vi "Lockin to DAQ SMO config.vi"(8 "error in (no error)":errorcluster, 9 "SamplingInfo":cluster{"Fs":dbl, "#S":i32}={"Fs"=1000.0, "#S"=1000}, 10 "AO Configuration":T7, 11 "AI Configuration":T10) -> (0 "error out":errorcluster, 2 "DAQ_Manager.setDAQConfig":T1 {"DAQmx.AI.config"."input terminal configuration" items=["default"=-1, "RSE"=10083, "NRSE"=10078, "Differential"=10106, "Pseudodifferential"=12529]; "DAQmx.AI.config"."AI.Coupling" items=["AC"=10045, "DC"=10050, "GND"=10066]; "DAQmx.AO.config"."output terminal configuration" items=["Default"=-1, "RSE"=10083, "Differential"=10106, "Pseudodifferential"=12529]})   [LabVIEW 2019]
uses:
  SMOs/DAQmx.AI/Typedefs/AI.Terminal-enum.ctl
  SMOs/DAQmx.AO/Typedefs/AO.Terminal-enum.ctl
  SMOs/DAQmx.AI/Typedefs/AI.Coupling-enum.ctl
  SMOs/DAQmx.AO/Typedefs/DAQmx.AO_Config.ctl
  SMOs/DAQmx.AI/Typedefs/DAQmx.AI_Config.ctl
  SMOs/DAQ_Manager/Typedefs/PrivateEvents--DAQ_Manager.setDAQConfig.ctl
  Typedefs/446xAO-enum.ctl
  Typedefs/AO.config-cluster.ctl
  Typedefs/AO.config-array.ctl
  Typedefs/AI.coupling-enum.ctl
  Typedefs/446xAI-enum.ctl
  Typedefs/AI.config-cluster.ctl
  Typedefs/AI.config-array.ctl
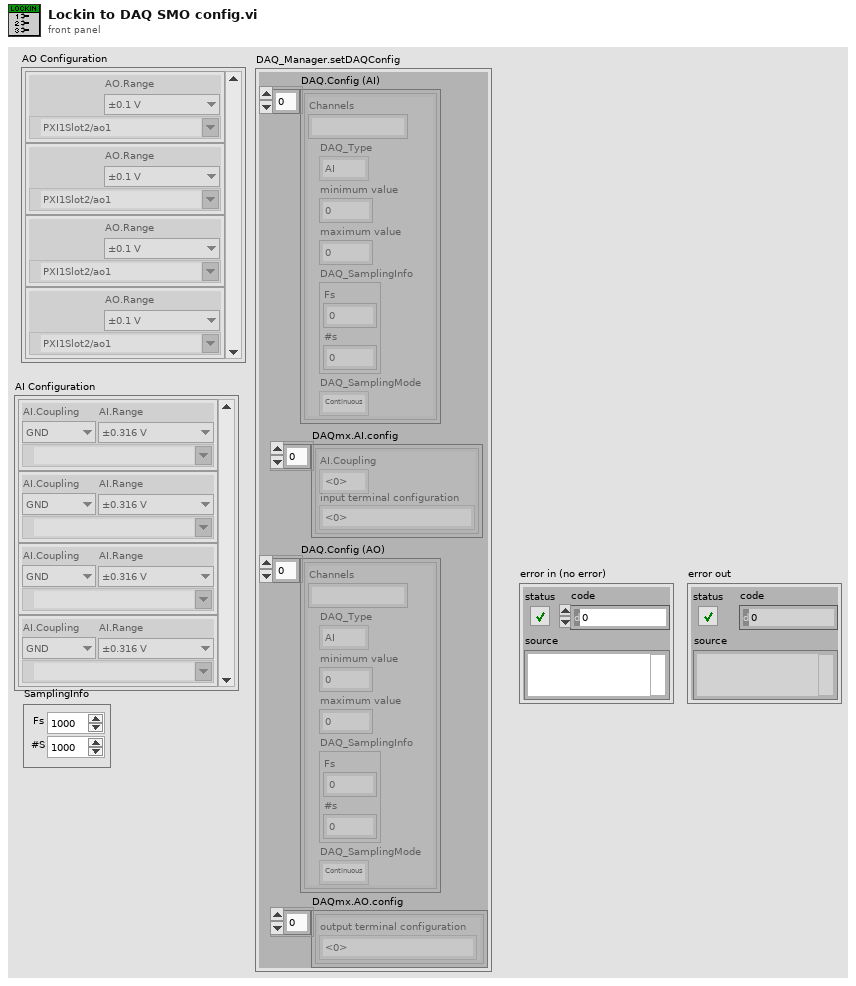
[diagram p1: front panel]
types:
  T1 = typedef "DAQ_Manager.lvclass/PrivateEvents--DAQ_Manager.setDAQConfig.ctl" = cluster{"DAQ.Config (AI)":cluster{"Channels":string, "DAQ_Type":enum16{"AI", "AO"}, "minimum value":dbl, "maximum value":dbl, "DAQ_SamplingInfo":cluster{"Fs":dbl, "#s":i32}, "DAQ_SamplingMode":enum16{"Continuous", "Finite"}}[], "DAQmx.AI.config":T2[], "DAQ.Config (AO)":cluster{"Channels":string, "DAQ_Type":enum16{"AI", "AO"}, "minimum value":dbl, "maximum value":dbl, "DAQ_SamplingInfo":cluster{"Fs":dbl, "#s":i32}, "DAQ_SamplingMode":enum16{"Continuous", "Finite"}}[], "DAQmx.AO.config":T5[]}
  T2 = typedef "DAQmx.AI.lvclass/DAQmx.AI_Config.ctl" = cluster{"AI.Coupling":T3, "input terminal configuration ":T4}
  T3 = typedef "DAQmx.AI.lvclass/AI.Coupling-enum.ctl" = i32
  T4 = typedef "DAQmx.AI.lvclass/AI.Terminal-enum.ctl" = i32
  T5 = typedef "DAQmx.AO.lvclass/DAQmx.AO_Config.ctl" = cluster{"output terminal configuration":T6}
  T6 = typedef "DAQmx.AO.lvclass/AO.Terminal-enum.ctl" = i32
  T7 = typedef "AO.config-array.ctl" = T8[]
  T8 = typedef "AO.config-cluster.ctl" = cluster{"AO.Range":T9, "AO.channels":tag}
  T9 = typedef "446xAO-enum.ctl" = enum16{"±0.1 V", "±1.0 V", "±10.0 V"}
  T10 = typedef "AI.config-array.ctl" = T11[]
  T11 = typedef "AI.config-cluster.ctl" = cluster{"AI.Coupling":T12, "AI.channels":tag, "AI.Range":T13}
  T12 = typedef "AI.coupling-enum.ctl" = enum16{"AC", "DC", "GND"}
  T13 = typedef "446xAI-enum.ctl" = enum16{"±0.316 V", "±1.00 V", "±3.16 V", "±10.0 V", "±31.6 V", "±42.4 V"}
  T14 = cluster{"Channels":string, "DAQ_Type":enum16{"AI", "AO"}, "minimum value":dbl, "maximum value":dbl, "DAQ_SamplingInfo":cluster{"Fs":dbl, "#s":i32}, "DAQ_SamplingMode":enum16{"Continuous", "Finite"}}[]
  T15 = cluster{"Channels":string, "DAQ_Type":enum16{"AI", "AO"}, "minimum value":dbl, "maximum value":dbl, "DAQ_SamplingInfo":cluster{"Fs":dbl, "#s":i32}, "DAQ_SamplingMode":enum16{"Continuous", "Finite"}}
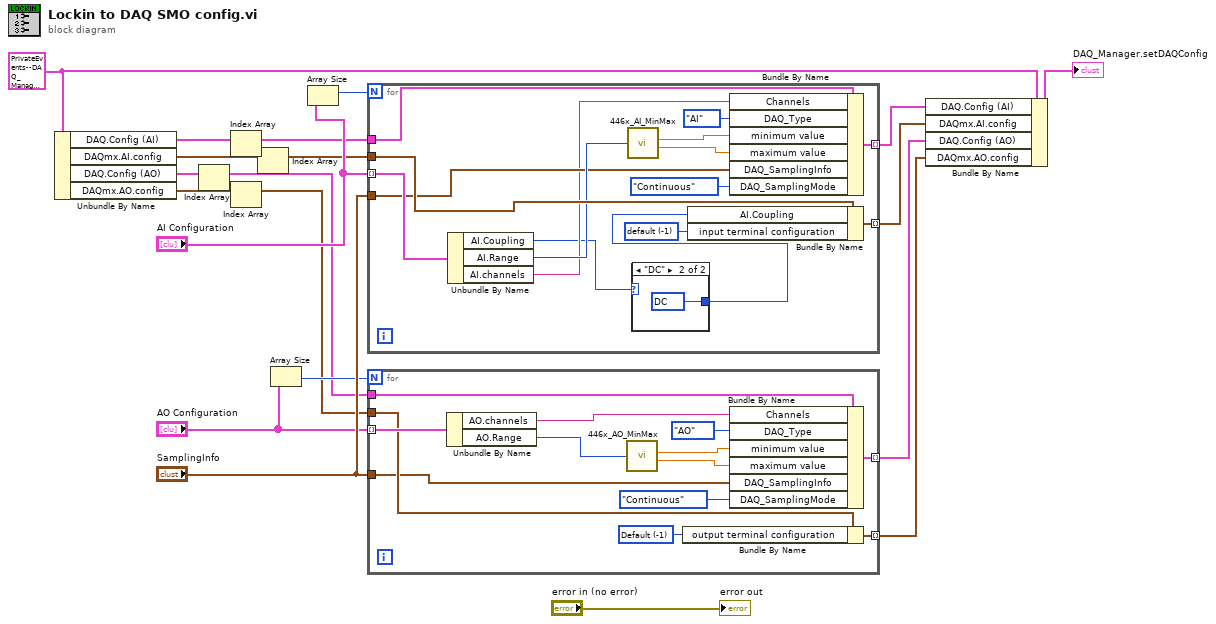
[diagram p0: block diagram]
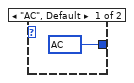
[diagram p2: hidden frame]
diagram:
  w2 = T1 {"DAQ.Config (AI)"=[{"Channels"="", "DAQ_Type"=enum."AI", "minimum value"=0.0, "maximum value"=0.0, "DAQ_SamplingInfo"={"Fs"=0.0, "#s"=0}, "DAQ_SamplingMode"=enum."Continuous"}], "DAQmx.AI.config"=[{"AI.Coupling"=10045, "input terminal configuration "=-1}], "DAQ.Config (AO)"=[{"Channels"="", "DAQ_Type"=enum."AI", "minimum value"=0.0, "maximum value"=0.0, "DAQ_SamplingInfo"={"Fs"=0.0, "#s"=0}, "DAQ_SamplingMode"=enum."Continuous"}], "DAQmx.AO.config"=[{"output terminal configuration"=-1}]} ("DAQ_Manager.setDAQConfig")
  n1 = Unbundle By Name(w2) -> ("DAQ.Config (AI)"=w17:T14, "DAQmx.AI.config"=w18:T2[], "DAQ.Config (AO)"=w19:T14, "DAQmx.AO.config"=w20:T5[])
  n2 = Index Array(array=w19) -> (element=w3:T15)  [unwired: 1 in]
  n3 = Index Array(array=w17) -> (element=w6:T15)  [unwired: 1 in]
  n4 = Index Array(array=w20) -> (element=w4:T5)  [unwired: 1 in]
  n5 = Index Array(array=w18) -> (element=w5:T2)  [unwired: 1 in]
  n6 = Array Size(array="AO Configuration") -> (size(s)=w9:i32)
  n7 = Array Size(array="AI Configuration") -> (size(s)=w7:i32)
  n8 = for {
    N: w7 -> [_]
    tunnel: w6 -> [w34]
    tunnel: w5 -> [w33]
    tunnel: "AI Configuration" -> [w35] mode=indexing
    tunnel: "SamplingInfo" -> [w28]
    tunnel: [w24] -> w14 mode=indexing
    tunnel: [w23] -> w13 mode=indexing
    w30 = T4 -1 items=["default"=-1, "RSE"=10083, "NRSE"=10078, "Differential"=10106, "Pseudodifferential"=12529] ("input terminal configuration")
    n9 = Unbundle By Name(w35) -> ("AI.Coupling"=w22:T12, "AI.Range"=w31:T13, "AI.channels"=w26:tag)
    n10 = call "446x_AI_MinMax.vi"("446x AI"=w31) -> ("AI.Min"=w32:dbl, "AI.Max"=w25:dbl)  [unwired: 6 in]
    n11 = case shown="\"DC\"" w22 {
      tunnel: [w36 w37] -> w21
      frame "AC", Default {
        w36 = T3 10045 items=["AC"=10045, "DC"=10050, "GND"=10066] ("AI.Coupling")
      }
      frame "DC" {
        w37 = T3 10050 items=["AC"=10045, "DC"=10050, "GND"=10066] ("AI.Coupling")
      }
    }
    n12 = Bundle By Name(cluster=w33, "AI.Coupling"=w21, "input terminal configuration"=w30) -> (w23:T2)
    n13 = Bundle By Name(cluster=w34, "Channels"=w26, "DAQ_Type"=enum16{"AI", "AO"}."AI", "minimum value"=w32, "maximum value"=w25, "DAQ_SamplingInfo"=w28, "DAQ_SamplingMode"=enum16{"Continuous", "Finite"}."Continuous") -> (w24:T15)
  }
  n14 = for {
    N: w9 -> [_]
    tunnel: w3 -> [w49]
    tunnel: w4 -> [w48]
    tunnel: "AO Configuration" -> [w50] mode=indexing
    tunnel: "SamplingInfo" -> [w45]
    tunnel: [w40] -> w12 mode=indexing
    tunnel: [w39] -> w11 mode=indexing
    w47 = T6 -1 items=["Default"=-1, "RSE"=10083, "Differential"=10106, "Pseudodifferential"=12529] ("output terminal configuration")
    n15 = Unbundle By Name(w50) -> ("AO.channels"=w41:tag, "AO.Range"=w38:T9)
    n16 = call "446x_AO_MinMax.vi"("AO.Range"=w38) -> ("AO.min"=w43:dbl, "AO.max"=w42:dbl)  [unwired: 6 in]
    n17 = Bundle By Name(cluster=w48, "output terminal configuration"=w47) -> (w39:T5)
    n18 = Bundle By Name(cluster=w49, "Channels"=w41, "DAQ_Type"=enum16{"AI", "AO"}."AO", "minimum value"=w43, "maximum value"=w42, "DAQ_SamplingInfo"=w45, "DAQ_SamplingMode"=enum16{"Continuous", "Finite"}."Continuous") -> (w40:T15)
  }
  n19 = Bundle By Name(cluster=w2, "DAQ.Config (AI)"=w14, "DAQmx.AI.config"=w13, "DAQ.Config (AO)"=w12, "DAQmx.AO.config"=w11) -> (→"DAQ_Manager.setDAQConfig":T1)
  "error out" <- "error in (no error)"
